vi "wash perispump.vi"(11 "channel":i8) -> ()   [LabVIEW 2023]
uses:
  <vilib>/DAQmx/create/channels.llb/DAQmx Create Channel (DI-Digital Input).vi
  <vilib>/DAQmx/read.llb/DAQmx Read (Digital 1D Bool 1Chan 1Samp).vi
panel:
  out "sensor":bool[](array[boolean])
  in  "stop":bool
  out "channel":string
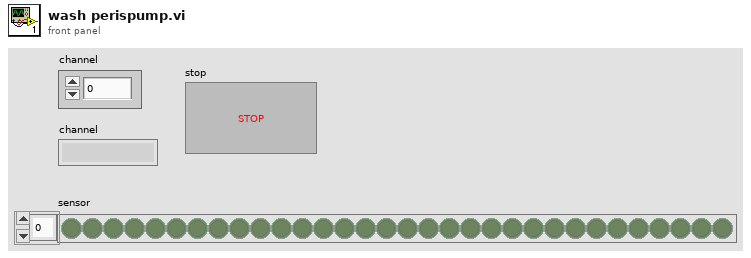
[diagram p1: front panel]
types:
  T1 = enum16{"Initialize", "Absolute Position", "Relative Pickup", "Relative Dispense", "Swich valve", "Bypass"}
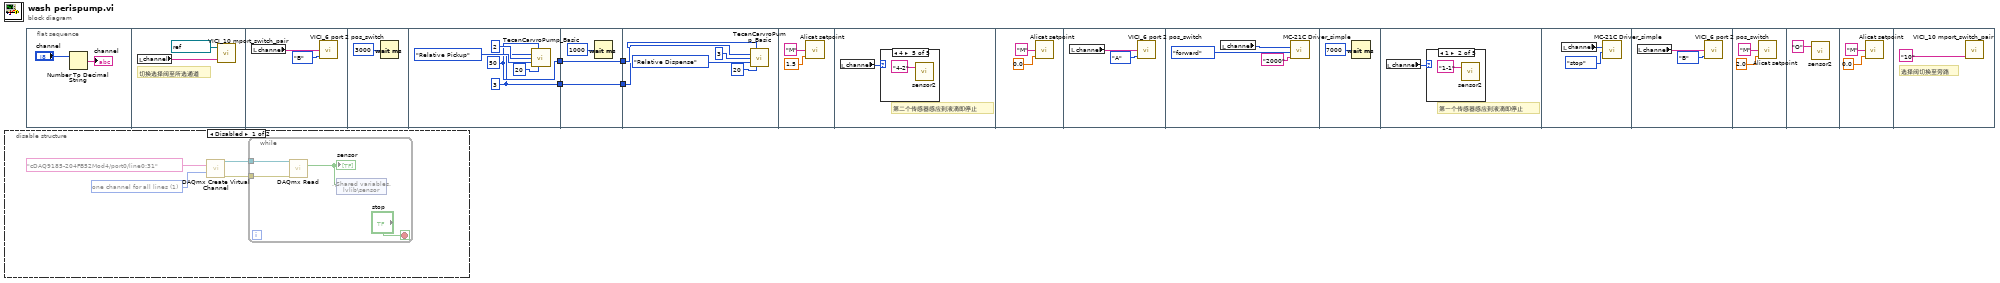
[diagram p0: block diagram]
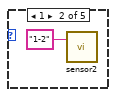
[diagram p4: hidden frame]
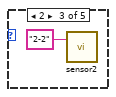
[diagram p5: hidden frame]
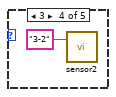
[diagram p6: hidden frame]
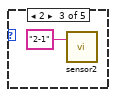
[diagram p8: hidden frame]
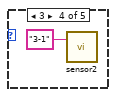
[diagram p9: hidden frame]
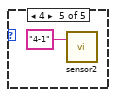
[diagram p10: hidden frame]
diagram:
  n1 = disable-structure shown="Disabled" {
    frame Disabled {
      w8 = 1 items=["one channel for each line", "one channel for all lines"] ("line grouping")
      n2 = call-poly <vilib>:"DAQmx Create Virtual Channel.vi"("lines"=tag "cDAQ9185-204FB52Mod4/port0/line0:31", "line grouping"=w8) -> ("task out"=w7:refnum<k21>, "error out"=w6:errorcluster)  [unwired: 12 in]
      n3 = while {
        tunnel: w7 -> [w12]
        tunnel: w6 -> [w11]
        stop <- "stop" stop-if-true
        n4 = call-poly <vilib>:"DAQmx Read.vi"("task/channels in"=w12, "error in"=w11) -> ("data"=w10:bool[])  [unwired: 11 in, 2 out]
        "sensor" <- w10
        n5 = shared-variable ".\\Shared variables.lvlib\\sensor"(w10) -> ()  [unwired: 1 in, 1 out]
      }
    }
    frame Enabled {
    }
  }
  n6 = flat-sequence {
    tunnel: [w21] -> w3
    tunnel: [w20] -> w1
    tunnel: [w27] -> w4
    tunnel: w3 -> [w27]
    tunnel: [w25] -> w2
    tunnel: w1 -> [w25]
    tunnel: w4 -> [w29]
    tunnel: w2 -> [w28]
    frame #0 {
      n7 = Number To Decimal String(number="channel") -> (decimal integer string=→"channel":string)  [unwired: 1 in]
    }
    frame #1 {
      # "切换选择阀至所选通道"
      n8 = local read "channel"() -> (w16:string)
      n9 = call "VICI_10 mport_switch_pair.vi"("Go to position"=w16, "Valve COM"=refnum<visa-resource-name> "COM8") -> ()  [unwired: 2 in, 1 out]
    }
    frame #2 {
      n10 = local read "channel"() -> (w17:string)
      n11 = call "VICI_6 port 2 pos_switch.vi"("Switch to position (A/B)"=enum16{"A", "B"}."B", "Valve ID"=w17) -> ()  [unwired: 2 in, 1 out]
    }
    frame #3 {
      n12 = Wait (ms)(milliseconds to wait=u32 3000) -> ()  [unwired: 1 out]
    }
    frame #4 {
      w21 = u16 50 ("Volume (μL)")
      w20 = u8 3 ("TecanPump address")
      n13 = call "TecanCarvroPump_Basic.vi"("Volume (μL)"=w21, "TecanPump address"=w20, "Valve"=u8 2, "Mode"=T1."Relative Pickup", "Speed (μL/s)"=u16 20) -> ()  [unwired: 10 in, 1 out]
    }
    frame #5 {
      n14 = Wait (ms)(milliseconds to wait=u32 1000) -> ()  [unwired: 1 out]
    }
    frame #6 {
      n15 = call "TecanCarvroPump_Basic.vi"("Volume (μL)"=w29, "TecanPump address"=w28, "Valve"=u8 3, "Mode"=T1."Relative Dispense", "Speed (μL/s)"=u16 20) -> ()  [unwired: 10 in, 1 out]
    }
    frame #7 {
      n16 = call "Alicat setpoint.vi"("Setpoint"=1.5, "Unit ID"="M") -> ()  [unwired: 3 in]
    }
    frame #8 {
      # "第二个传感器感应到液滴即停止"
      n17 = local read "channel"() -> (w35:i8)
      n18 = case shown="4" w35 {
        frame 0, Default {
        }
        frame 1 {
          n19 = call "sensor2.vi"("Sensor"="1-2") -> ()  [unwired: 1 in, 2 out]
        }
        frame 2 {
          n20 = call "sensor2.vi"("Sensor"="2-2") -> ()  [unwired: 1 in, 2 out]
        }
        frame 3 {
          n21 = call "sensor2.vi"("Sensor"="3-2") -> ()  [unwired: 1 in, 2 out]
        }
        frame 4 {
          n22 = call "sensor2.vi"("Sensor"="4-2") -> ()  [unwired: 1 in, 2 out]
        }
      }
    }
    frame #9 {
      n23 = call "Alicat setpoint.vi"("Setpoint"=0.0, "Unit ID"="M") -> ()  [unwired: 3 in]
    }
    frame #10 {
      n24 = local read "channel"() -> (w43:string)
      n25 = call "VICI_6 port 2 pos_switch.vi"("Switch to position (A/B)"=enum16{"A", "B"}."A", "Valve ID"=w43) -> ()  [unwired: 2 in, 1 out]
    }
    frame #11 {
      n26 = local read "channel"() -> (w46:i8)
      n27 = call "MC-21C Driver_simple.vi"("Step"="2000", "Operation"=enum16{"forward", "backward", "stop"}."forward", "Address"=w46) -> ()  [unwired: 8 in, 1 out]
    }
    frame #12 {
      n28 = Wait (ms)(milliseconds to wait=u32 7000) -> ()  [unwired: 1 out]
    }
    frame #13 {
      # "第一个传感器感应到液滴即停止"
      n29 = local read "channel"() -> (w48:i8)
      n30 = case shown="1" w48 {
        frame 0, Default {
        }
        frame 1 {
          n31 = call "sensor2.vi"("Sensor"="1-1") -> ()  [unwired: 1 in, 2 out]
        }
        frame 2 {
          n32 = call "sensor2.vi"("Sensor"="2-1") -> ()  [unwired: 1 in, 2 out]
        }
        frame 3 {
          n33 = call "sensor2.vi"("Sensor"="3-1") -> ()  [unwired: 1 in, 2 out]
        }
        frame 4 {
          n34 = call "sensor2.vi"("Sensor"="4-1") -> ()  [unwired: 1 in, 2 out]
        }
      }
    }
    frame #14 {
      n35 = local read "channel"() -> (w53:i8)
      n36 = call "MC-21C Driver_simple.vi"("Operation"=enum16{"forward", "backward", "stop"}."stop", "Address"=w53) -> ()  [unwired: 9 in, 1 out]
    }
    frame #15 {
      n37 = local read "channel"() -> (w56:string)
      n38 = call "VICI_6 port 2 pos_switch.vi"("Switch to position (A/B)"=enum16{"A", "B"}."B", "Valve ID"=w56) -> ()  [unwired: 2 in, 1 out]
    }
    frame #16 {
      n39 = call "Alicat setpoint.vi"("Setpoint"=2.0, "Unit ID"="M") -> ()  [unwired: 3 in]
    }
    frame #17 {
      n40 = call "sensor2.vi"("Sensor"="O") -> ()  [unwired: 1 in, 2 out]
    }
    frame #18 {
      n41 = call "Alicat setpoint.vi"("Setpoint"=0.0, "Unit ID"="M") -> ()  [unwired: 3 in]
    }
    frame #19 {
      # "选择阀切换至旁路"
      n42 = call "VICI_10 mport_switch_pair.vi"("Go to position"="10") -> ()  [unwired: 3 in, 1 out]
    }
  }
